vi "TeamNumberChange.vi"(0 "String in":string) -> (7 "String out":string)   [LabVIEW 2015]
uses:
  Global Data.vi
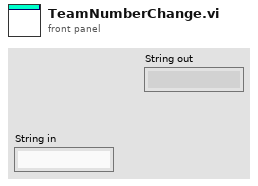
[diagram p1: front panel]
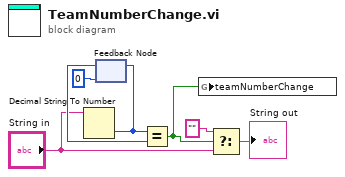
[diagram p0: block diagram]
diagram:
  n1 = Decimal String To Number(string="String in") -> (number=w5:i32)  [unwired: 2 in, 1 out]
  n2 = feedback #1(0) -> (w7:i32)
  n3 = feedback-in #1(w5) -> ()
  n4 = Equal?(x=w5, y=w7) -> (x = y?=w1:bool)
  n5 = global write "Global Data.vi" "teamNumberChange"(w1) -> ()
  n6 = Select(t="", s=w1, f="String in") -> (s? t:f=→"String out":string)
